vi "Mean.vi"   [LabVIEW 2017, in "NI_AALBase.lvlib"]
doc: "Computes the <B>mean</B> of the values in the input sequence <B>X</B>. You must manually select the polymorphic instance you want to use."
uses:
  <vilib>/Analysis/NI_AALBase.lvlib
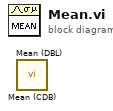
[diagram p0: block diagram]
diagram:
  n1 = call <vilib>:"Mean (CDB).vi"() -> ()  [unwired: 1 in, 2 out]
  n2 = call <vilib>:"Mean (DBL).vi"() -> ()  [unwired: 1 in, 2 out]
